vi "correlations.vi"() -> ()   [LabVIEW 2023]
uses:
  <vilib>/Analysis/2dsp.llb/1D Cross Correlation (DBL).vi
  <vilib>/Analysis/NI_AALPro.lvlib
  <vilib>/measure/NI_MABase.lvlib
panel:
  out "output waveform":waveform(dbl)(graph)
  out "signal out":waveform(dbl)(graph)
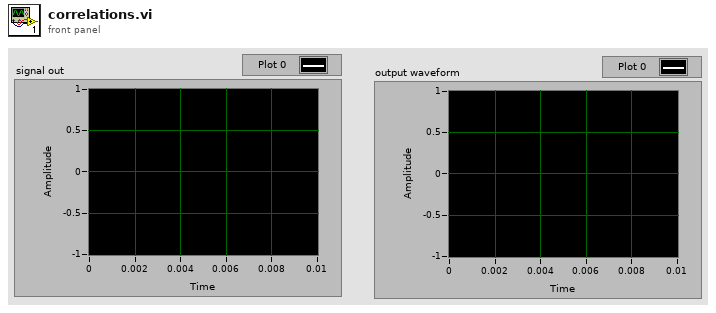
[diagram p1: front panel]
types:
  T1 = enum16{"Sine Wave", "Triangle Wave", "Square Wave", "Sawtooth Wave"}
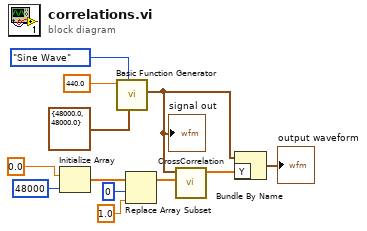
[diagram p0: block diagram]
diagram:
  n1 = Initialize Array(0.0 ("element"), 48000 ("dimension size")) -> (w7:dbl[])
  n2 = call <vilib>:"Basic Function Generator.vi"("sampling info"=cluster{"Fs":dbl, "#s":dbl} {"Fs"=48000.0, "#s"=48000.0}, "signal type"=T1."Sine Wave", "frequency"=440.0) -> ("signal out"=w3:waveform(dbl))  [unwired: 6 in, 2 out]
  "signal out" <- w3
  n3 = Replace Array Subset(array=w7, new element=1.0 ("new element/subarray"), index=0) -> (w4:dbl[])
  n4 = call-poly <vilib>:"CrossCorrelation.vi"("Y"=w4, "X"=w3) -> ("Rxy"=w2:dbl[])  [unwired: 8 in, 1 out]
  n5 = Bundle By Name(cluster=w3, "Y"=w2) -> (→"output waveform":waveform(dbl))
